vi "initialise.vi"(8 "error in (no error)":errorcluster, 11 "GenericPlugin in":refnum<class "ScanHeadAK130114ResonanceFlexRIO.lvclass">) -> (0 "error out":errorcluster, 3 "GenericPlugin out":refnum<class "ScanHeadAK130114ResonanceFlexRIO.lvclass">)   [LabVIEW 2010, in "ScanHeadAK130114ResonanceFlexRIO.lvclass"]
doc: "The dynamic dispatch-version of this VI initalises the plug-in object by allocating and initalising any dynamic resources need."
uses:
  ScanHeadAK130114ResonanceFlexRIO.lvclass
  GenericScanHead/GenericScanHead/GenericScanHead.lvclass
  SignalWriter/GenericSignalWriter/GenericSignalWriter/GenericSignalWriter.lvclass
  AnalogOut/GenericAnalogOut/GenericAnalogOut/GenericAnalogOut.lvclass
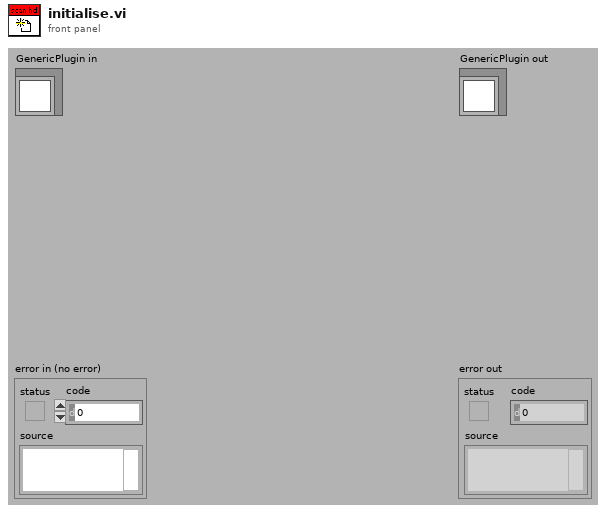
[diagram p1: front panel]
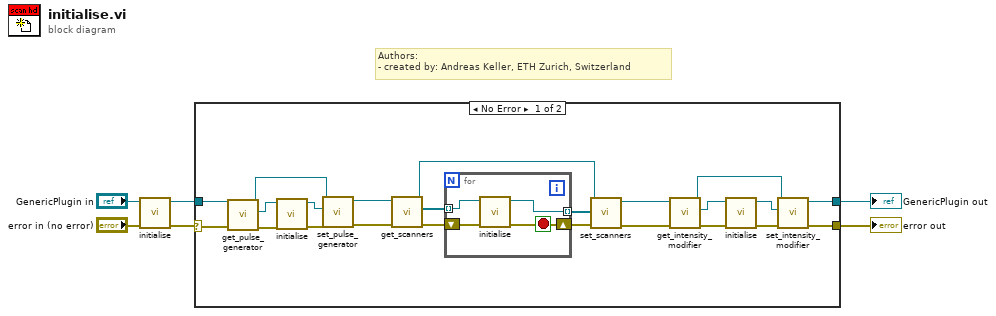
[diagram p0: block diagram]
diagram:
  # "Authors: \n- created by: Andreas Keller, ETH Zurich, Switzerland"
  n1 = call-parent "initialise.vi"("error in (no error)"="error in (no error)", "GenericPlugin in"="GenericPlugin in") -> ("error out"=w4:errorcluster, "GenericPlugin out"=w3:refnum<class "ScanHeadAK130114ResonanceFlexRIO.lvclass">)  [unwired: 8 in]
  n2 = case shown="No Error" w4 {
    selector: w4 -> [w29 w35]
    tunnel: w3 -> [w23 w34]
    tunnel: [w12 w35] -> w2
    tunnel: [w9 w34] -> w1
    frame No Error {
      n3 = call-dynamic "get_pulse_generator.vi"("error in (no error)"=w29, "ScanHeadAK130114ResonanceFlexRIO in"=w23) -> ("error out"=w28:errorcluster, "pulse generator"=w27:refnum<class "GenericSignalWriter.lvclass">, "ScanHeadAK130114ResonanceFlexRIO out"=w24:refnum<class "ScanHeadAK130114ResonanceFlexRIO.lvclass">)  [unwired: 7 in]
      n4 = call-dynamic "initialise.vi"("error in (no error)"=w28, "GenericPlugin in"=w27) -> ("error out"=w26:errorcluster, "GenericPlugin out"=w25:refnum<class "GenericSignalWriter.lvclass">)  [unwired: 8 in]
      n5 = call-dynamic "set_pulse_generator.vi"("error in (no error)"=w26, "pulse generator"=w25, "ScanHeadAK130114ResonanceFlexRIO in"=w24) -> ("error out"=w22:errorcluster, "ScanHeadAK130114ResonanceFlexRIO out"=w21:refnum<class "ScanHeadAK130114ResonanceFlexRIO.lvclass">)  [unwired: 7 in]
      n6 = call-dynamic "get_scanners.vi"("error in (no error)"=w22, "ScanHeadAK130114ResonanceFlexRIO in"=w21) -> ("error out"=w19:errorcluster, "scanners"=w18:refnum<class "GenericSignalWriter.lvclass">[], "ScanHeadAK130114ResonanceFlexRIO out"=w20:refnum<class "ScanHeadAK130114ResonanceFlexRIO.lvclass">)  [unwired: 7 in]
      n7 = for {
        shift-right: [w30] -> w16
        shift-left: w19 -> [w31]
        tunnel: w18 -> [w33] mode=indexing
        tunnel: [w32] -> w17 mode=indexing
        stop <- w30 stop-if-true
        n8 = call-dynamic "initialise.vi"("error in (no error)"=w31, "GenericPlugin in"=w33) -> ("error out"=w30:errorcluster, "GenericPlugin out"=w32:refnum<class "GenericSignalWriter.lvclass">)  [unwired: 8 in]
      }
      n9 = call-dynamic "set_scanners.vi"("error in (no error)"=w16, "scanners"=w17, "ScanHeadAK130114ResonanceFlexRIO in"=w20) -> ("error out"=w15:errorcluster, "ScanHeadAK130114ResonanceFlexRIO out"=w7:refnum<class "ScanHeadAK130114ResonanceFlexRIO.lvclass">)  [unwired: 7 in]
      n10 = call-dynamic "get_intensity_modifier.vi"("error in (no error)"=w15, "ScanHeadAK130114ResonanceFlexRIO in"=w7) -> ("error out"=w14:errorcluster, "intensity modifier"=w11:refnum<class "GenericAnalogOut.lvclass">, "ScanHeadAK130114ResonanceFlexRIO out"=w10:refnum<class "ScanHeadAK130114ResonanceFlexRIO.lvclass">)  [unwired: 7 in]
      n11 = call-dynamic "initialise.vi"("error in (no error)"=w14, "GenericPlugin in"=w11) -> ("error out"=w13:errorcluster, "GenericPlugin out"=w8:refnum<class "GenericAnalogOut.lvclass">)  [unwired: 8 in]
      n12 = call-dynamic "set_intensity_modifier.vi"("error in (no error)"=w13, "intensity modifier"=w8, "ScanHeadAK130114ResonanceFlexRIO in"=w10) -> ("error out"=w12:errorcluster, "ScanHeadAK130114ResonanceFlexRIO out"=w9:refnum<class "ScanHeadAK130114ResonanceFlexRIO.lvclass">)  [unwired: 7 in]
    }
    frame Error {
    }
  }
  "error out" <- w2
  "GenericPlugin out" <- w1
